vi "ControlEnhanced.vi"() -> ()   [LabVIEW 2018]
uses:
  <vilib>/Platform/TimedLoop/XDataNode/timing_clust.ctl
  <vilib>/Platform/TimedLoop/XDataNode/nitl_modes.ctl
  <vilib>/Platform/TimedLoop/XDataNode/wakeup.ctl
  <vilib>/myRIO/Instrument Drivers/Onboard IO/AI/typedefs/AI Reference.ctl
  <vilib>/myRIO/Common/Instrument Driver Framework/Utilities/typedefs/myRIO Generic Hardware Reference.ctl
  <vilib>/myRIO/Common/Instrument Driver Framework/Utilities/typedefs/Hardware Version Enum.ctl
  <vilib>/myRIO/Common/Instrument Driver Framework/Utilities/typedefs/myRIO v1.0 Reference.ctl
  <vilib>/myRIO/Common/Instrument Driver Framework/Utilities/typedefs/Generic FPGA Reference.ctl
  <vilib>/myRIO/Common/Instrument Driver Framework/myRIO v1.0/AI/typedefs/AI Channels List.ctl
  <vilib>/myRIO/Common/Instrument Driver Framework/myRIO v1.0/AI/typedefs/AI Channels Enum.ctl
  <vilib>/myRIO/Common/Instrument Driver Framework/Utilities/typedefs/Analog Scaling Constants List.ctl
  <vilib>/myRIO/Common/Instrument Driver Framework/Utilities/typedefs/Analog Scaling Constants.ctl
  <vilib>/userdefined/High Color/nirio_resource_hc.ctl
  <vilib>/myRIO/Instrument Drivers/Onboard IO/AO/typedefs/AO Reference.ctl
  <vilib>/myRIO/Common/Instrument Driver Framework/myRIO v1.0/AO/typedefs/AO Channels List.ctl
  <vilib>/myRIO/Common/Instrument Driver Framework/myRIO v1.0/AO/typedefs/AO Channels Enum.ctl
  <vilib>/myRIO/Common/Instrument Driver Framework/Utilities/vis/Is FPGA Ref Available.vi
  <vilib>/myRIO/Common/Instrument Driver Framework/myRIO v1.0/AI/vis/myRIO v1.1 Open AI.vi
  <vilib>/myRIO/Instrument Drivers/Onboard IO/AI/vis/Read.vi
  <vilib>/myRIO/Common/Instrument Driver Framework/myRIO v1.0/AO/vis/myRIO v1.1 Open AO.vi
  <vilib>/myRIO/Instrument Drivers/Onboard IO/AO/vis/Write.vi
  <vilib>/myRIO/Common/Instrument Driver Framework/myRIO v1.0/PWM/vis/myRIO v1.1 Open PWM.vi
  <vilib>/myRIO/Common/Instrument Driver Framework/Utilities/vis/Validate Channels.vi
  <vilib>/myRIO/Common/Instrument Driver Framework/myRIO v1.0/AI/vis/myRIO v1.0 Reserve AI.vi
  <vilib>/myRIO/Common/Instrument Driver Framework/myRIO v1.0/AO/vis/myRIO v1.0 Reserve AO.vi
  <vilib>/myRIO/Common/Instrument Driver Framework/myRIO v1.0/PWM/vis/myRIO v1.0 Reserve PWM.vi
  <vilib>/myRIO/Common/Instrument Driver Framework/myRIO v1.0/AI/vis/myRIO v1.0 Build MUX Configuration AI.vi
  <vilib>/myRIO/Common/Instrument Driver Framework/myRIO v1.0/Resource Manager/vis/myRIO v1.0 Reserve Channel List.vi
  <vilib>/myRIO/Common/Instrument Driver Framework/myRIO v1.0/AO/vis/myRIO v1.0 Build MUX Configuration AO.vi
  <vilib>/myRIO/Common/Instrument Driver Framework/myRIO v1.0/PWM/vis/myRIO v1.0 Build MUX Configuration PWM.vi
  <vilib>/myRIO/Common/Instrument Driver Framework/myRIO v1.0/Resource Manager/vis/myRIO v1.0 Reserve Channel.vi
  <vilib>/myRIO/Common/Instrument Driver Framework/myRIO v1.0/Resource Manager/vis/myRIO v1.0 Unreserve Channel.vi
  <vilib>/myRIO/Common/Instrument Driver Framework/myRIO v1.0/Resource Manager/vis/myRIO v1.0 Create Configuration List.vi
  <vilib>/myRIO/Common/Instrument Driver Framework/myRIO v1.0/Resource Manager/vis/myRIO v1.0 Build Mutex Name.vi
  <vilib>/Utility/VariantDataType/GetNumericInfo.vi
  <vilib>/Utility/error.llb/Error Cluster From Error Code.vi
  <vilib>/myRIO/Common/Instrument Driver Framework/myRIO v1.0/myRIO v1.1 Open.vi
  <vilib>/myRIO/Common/Instrument Driver Framework/myRIO v1.0/AI/vis/myRIO v1.0 Get Scaling Constants AI.vi
  <vilib>/myRIO/Common/Instrument Driver Framework/Utilities/vis/IO Manager.vi
  <vilib>/myRIO/Common/Instrument Driver Framework/Utilities/vis/Configuration Manager.vi
  <vilib>/myRIO/Common/Instrument Driver Framework/myRIO v1.0/myRIO v1.0 Close.vi
  <vilib>/myRIO/Common/Instrument Driver Framework/myRIO v1.0/AI/vis/myRIO v1.0 Read AI.vi
  <vilib>/myRIO/Common/Instrument Driver Framework/myRIO v1.0/AO/vis/myRIO v1.0 Get Scaling Constants AO.vi
  <vilib>/myRIO/Common/Instrument Driver Framework/myRIO v1.0/AO/vis/myRIO v1.0 Write AO.vi
  <vilib>/myRIO/Common/Instrument Driver Framework/myRIO v1.0/Resource Manager/vis/myRIO v1.0 Configure IO.vi
  <vilib>/myRIO/Common/Instrument Driver Framework/myRIO v1.0/PWM/vis/myRIO v1.0 Write PWM.vi
  <vilib>/platform/TimedLoop/XDataNode/XDataNode.xnode
  <vilib>/myRIO/Express VI/Onboard IO/AI/AI Express VI.xnode
  <vilib>/myRIO/Instrument Drivers/Onboard IO/AI/vis/myRIO AI Open.xnode
  <vilib>/myRIO/Express VI/Onboard IO/AO/AO Express VI.xnode
  <vilib>/myRIO/Instrument Drivers/Onboard IO/AO/vis/myRIO AO Open.xnode
  <vilib>/myRIO/Instrument Drivers/Onboard IO/AI/AI.lvlib
  <vilib>/myRIO/Instrument Drivers/Onboard IO/AO/AO.lvlib
  <vilib>/Platform/TimedLoop/XDataNode/XDNodeRunTimeDep.lvlib
  <vilib>/myRIO/Instrument Drivers/Onboard IO/PWM/PWM.lvlib
panel:
  in  "MAKE ACTUATOR EXPLODE":bool caption="Blank Button"
  out "FSR Voltage over Time":dbl(graph)
  in  "Stop Button":bool
  in  "Pressure \nSetpoint (kPa)":dbl(slide)=5.5 scale=0.0..30.0
  in  "PWM channel":tag="B/PWM0"
  in  "[ESC]":bool
  in  "Actuator Servo":dbl(slide) scale=-200.0..200.0
  in  "freq [Hz]":dbl=50.0
  out "pulse width [ms]":dbl=1.5
  out "duty cycle [%]":dbl
  in  "null offset":bool
  out "offset [%FS]":dbl
  in  "Button \nMode":bool
  out "bUTTON":bool
  out "Null Offset\n(Zero)":dbl
  in  "Ok":bool
  in  "Tolerance":dbl=0.5 format="%0.4f"
  in  "CRUSH IT":bool caption="Blank Button"
  in  "GRIP HARDER":bool caption="Blank Button"
  in  "GRIP":bool caption="Blank Button"
  in  "RELEASE":bool caption="Blank Button"
  in  "SoVal On/Off":bool
  in  "Gas Reg\n(Manual)":dbl(slide) scale=0.0..0.16
  in  "OK Button":bool
  in  "SELF-DESTRUCT BUTTON":bool
  in  "Operating Mode":string(combo)="1"
  in  "Upper \nBound":dbl=0.1 format="%#_13g"
  in  "Lower \nBound":dbl=0.04 format="%#_13g"
  in  "Signal Frequency / Hz":i64=200
  in  "Factor of Decrease":dbl=1e-05
  in  "Factor of Increase":dbl=1e-05
  out "SoVal":bool
  in  "BIGGER SELF-DESTRUCT BUTTON":bool
  out "SoVal\nSoVal (C/AO0 (AO0))":dbl
  out "Gas Reg. (A/AO0 (Pin 2))":dbl=0.04 min=0.04 max=0.1
  in  "Pressure \nSetpoint":dbl(slide)=5.5 scale=0.0..10.0
  out "Force Resistor kPa)":dbl
  out "FSR Dial (kPa)":dbl(knob) scale=-0.5..30.0
  out "PP 2":dbl
  out "PP Dial":dbl(knob) scale=-0.5..11.0
  out "PP":bool
  out "FSR":bool
  in  "PP Weight":dbl=0.1 min=0.0 max=1.0 step=0.001
  in  "FSR Weight":dbl=0.1 min=0.0 max=1.0 step=0.0001
  # "WARNING: it really does what it says."
  # "These are calculated based on the user-input lower and upper bounds. TODO: hide these buttons in automatic mode"
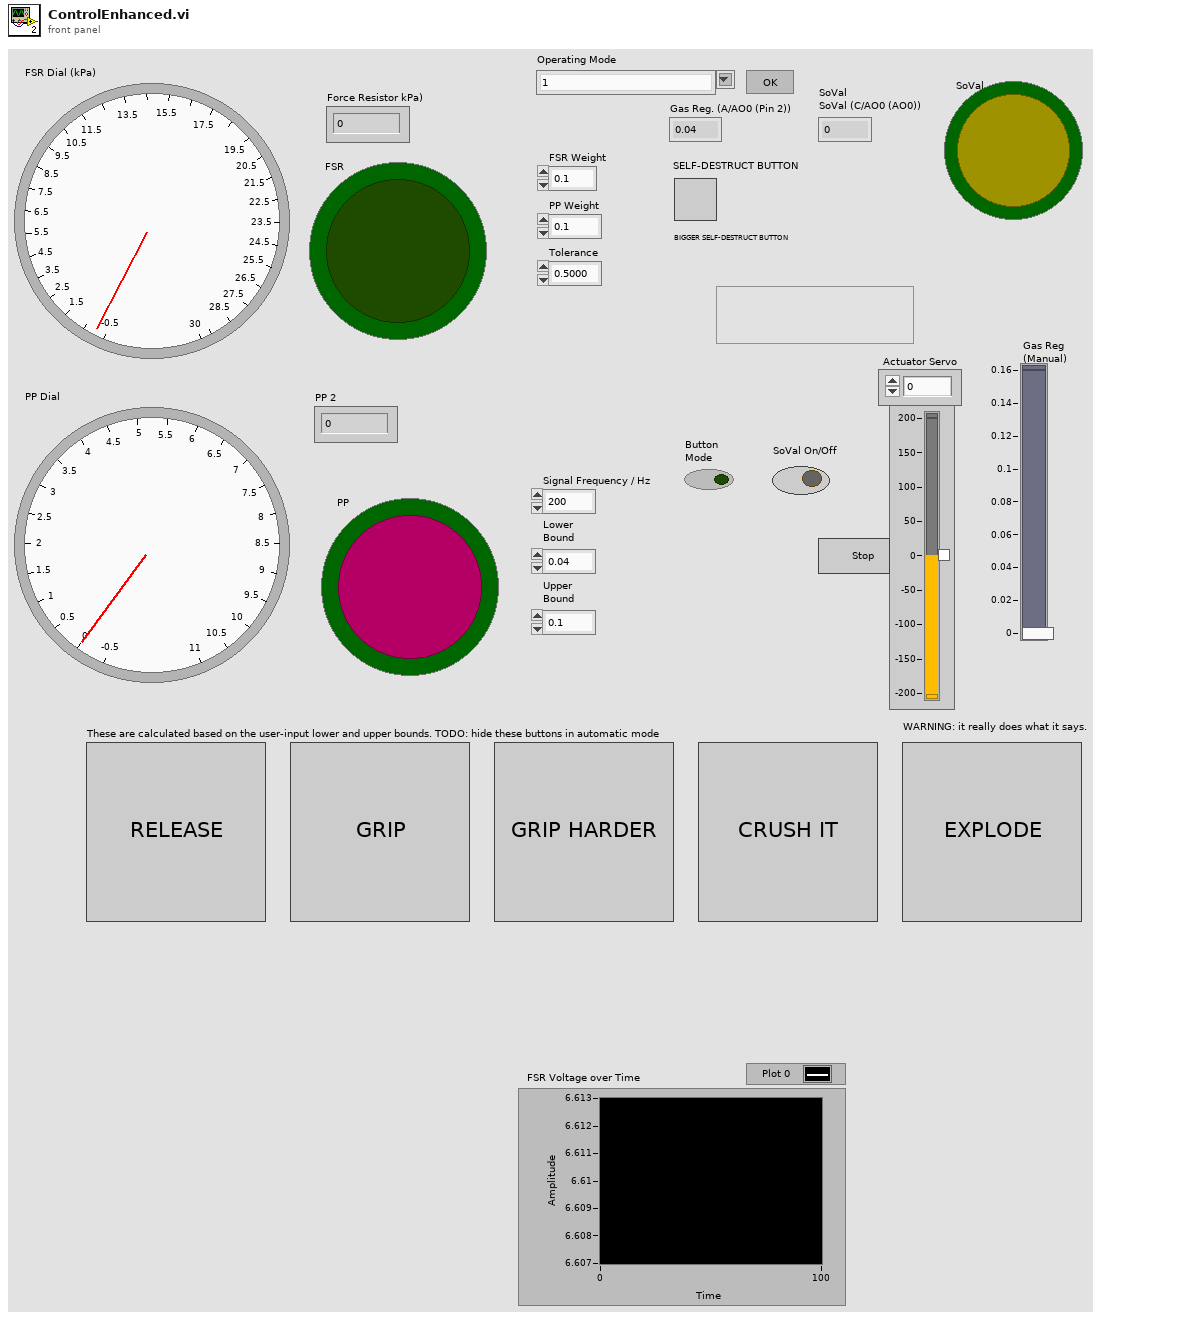
[diagram p1: front panel]
types:
  T1 = typedef "XDNodeRunTimeDep.lvlib/timing_clust.ctl" = cluster{"Expected End [f-1]":u64, "Actual End [f-1]":u64, "Finished Late? [f-1]":bool, "Expected End [i-1]":u64, "Actual End [i-1]":u64, "Finished Late? [i-1]":bool, "Expected Start [i]":u64, "Actual Start [i]":u64, "Expected Start [f]":u64, "Actual Start [f]":u64, "Source Name":string, "Structure Name":string, "Period":i64, "Deadline":i64, "Offset":i64, "Start":i64, "Priority":i32, "Timeout":i32, "Mode":T2, "Wakeup Reason":T3, "Error":errorcluster, "Source Type":string, "Secondary Source Type":string, "Global End Time":u64, "Global Start Time":u64, "Frame Duration":u64, "Iteration Duration":u64, "Assigned CPU":i32, "I/O Scan Engine Mode":u32}
  T2 = typedef "XDNodeRunTimeDep.lvlib/nitl_modes.ctl" = enum32{"No Change", "Process missed periods, maintain original phase", "Discard missed periods, maintain original phase", "Process missed periods, ignore original phase", "Discard missed periods, ignore original phase"}
  T3 = typedef "XDNodeRunTimeDep.lvlib/wakeup.ctl" = enum32{"Normal", "Aborted", "Asynchronous wakeup", "Timing source error", "Timed loop error", "Timeout"}
  T4 = typedef "AO.lvlib/AO Reference.ctl" = cluster{"myRIO Reference":T5, "AO Channel List":T9, "AO Scaling Constant List":T11}
  T5 = typedef "myRIO Generic Hardware Reference.ctl" = cluster{"myRIO Model":T6, "myRIO Hardware Reference":T7}
  T6 = typedef "Hardware Version Enum.ctl" = enum16{"Unknown", "myRIO-1900", "myRIO-1950", "roboRIO", "NI ELVIS RIO CM", "ELVIS III"}
  T7 = typedef "myRIO v1.0 Reference.ctl" = cluster{"Generic FPGA Reference":T8, "Allow multiple opens":bool}
  T8 = typedef "Generic FPGA Reference.ctl" = refnum<k20>
  T9 = typedef "AO Channels List.ctl" = T10[]
  T10 = typedef "AO Channels Enum.ctl" = enum16{"Not Connected", "AudioOut/Left", "AudioOut/Right", "C/AO0", "C/AO1", "A/AO0", "A/AO1", "B/AO0", "B/AO1"}
  T11 = typedef "Analog Scaling Constants List.ctl" = T12[]
  T12 = typedef "Analog Scaling Constants.ctl" = cluster{"LSB Weight (Volts)":dbl, "Offset (Volts)":dbl, "Signed?":bool}
  T13 = typedef "nirio_resource_hc.ctl" = tag
  T14 = typedef "AI.lvlib/AI Reference.ctl" = cluster{"myRIO Reference":T5, "AI Channels List":T15, "AI Scaling Constants List":T11}
  T15 = typedef "AI Channels List.ctl" = T16[]
  T16 = typedef "AI Channels Enum.ctl" = enum16{"Not Connected", "AudioIn/Left", "AudioIn/Right", "C/AI0", "C/AI1", "A/AI0", "A/AI1", "A/AI2", "A/AI3", "A/AI4", "A/AI5", "A/AI6", "A/AI7", "B/AI0", "B/AI1", "B/AI2", "B/AI3", "B/AI4", "B/AI5", "B/AI6", "B/AI7", "AI/AI0", "AI/AI1", "AI/AI2", "AI/AI3", "A/AI0 (DIFF)", "A/AI1 (DIFF)", "A/AI2 (DIFF)", "A/AI3 (DIFF)", "B/AI0 (DIFF)", "B/AI1 (DIFF)", "B/AI2 (DIFF)", "B/AI3 (DIFF)"}
  T17 = typedef "PWM.lvlib/PWM Reference.ctl" = cluster{"myRIO Reference":T5, "PWM Channels Enum":T18, "PWM Configuration":T19}
  T18 = typedef "PWM Channels Enum.ctl" = enum16{"Not Connected", "C/PWM0", "C/PWM1", "A/PWM0", "A/PWM1", "A/PWM2", "A/PWM3", "A/PWM4", "A/PWM5", "A/PWM6", "A/PWM7", "A/PWM8", "A/PWM9", "A/PWM10", "A/PWM11", "A/PWM12", "A/PWM13", "A/PWM14", "A/PWM15", "A/PWM16", "A/PWM17", "A/PWM18", "A/PWM19", "B/PWM0", "B/PWM1", "B/PWM2", "B/PWM3", "B/PWM4", "B/PWM5", "B/PWM6", "B/PWM7", "B/PWM8", "B/PWM9", "B/PWM10", "B/PWM11", "B/PWM12", "B/PWM13", "B/PWM14", "B/PWM15", "B/PWM16", "B/PWM17", "B/PWM18", "B/PWM19", "PWM/PWM0", "PWM/PWM1", "PWM/PWM2", "PWM/PWM3", "PWM/PWM4", "PWM/PWM5", "PWM/PWM6", "PWM/PWM7", "PWM/PWM8", "PWM/PWM9"}
  T19 = typedef "PWM.lvlib/PWM Configuration.ctl" = cluster{"Frequency":dbl, "Duty Cycle":dbl}
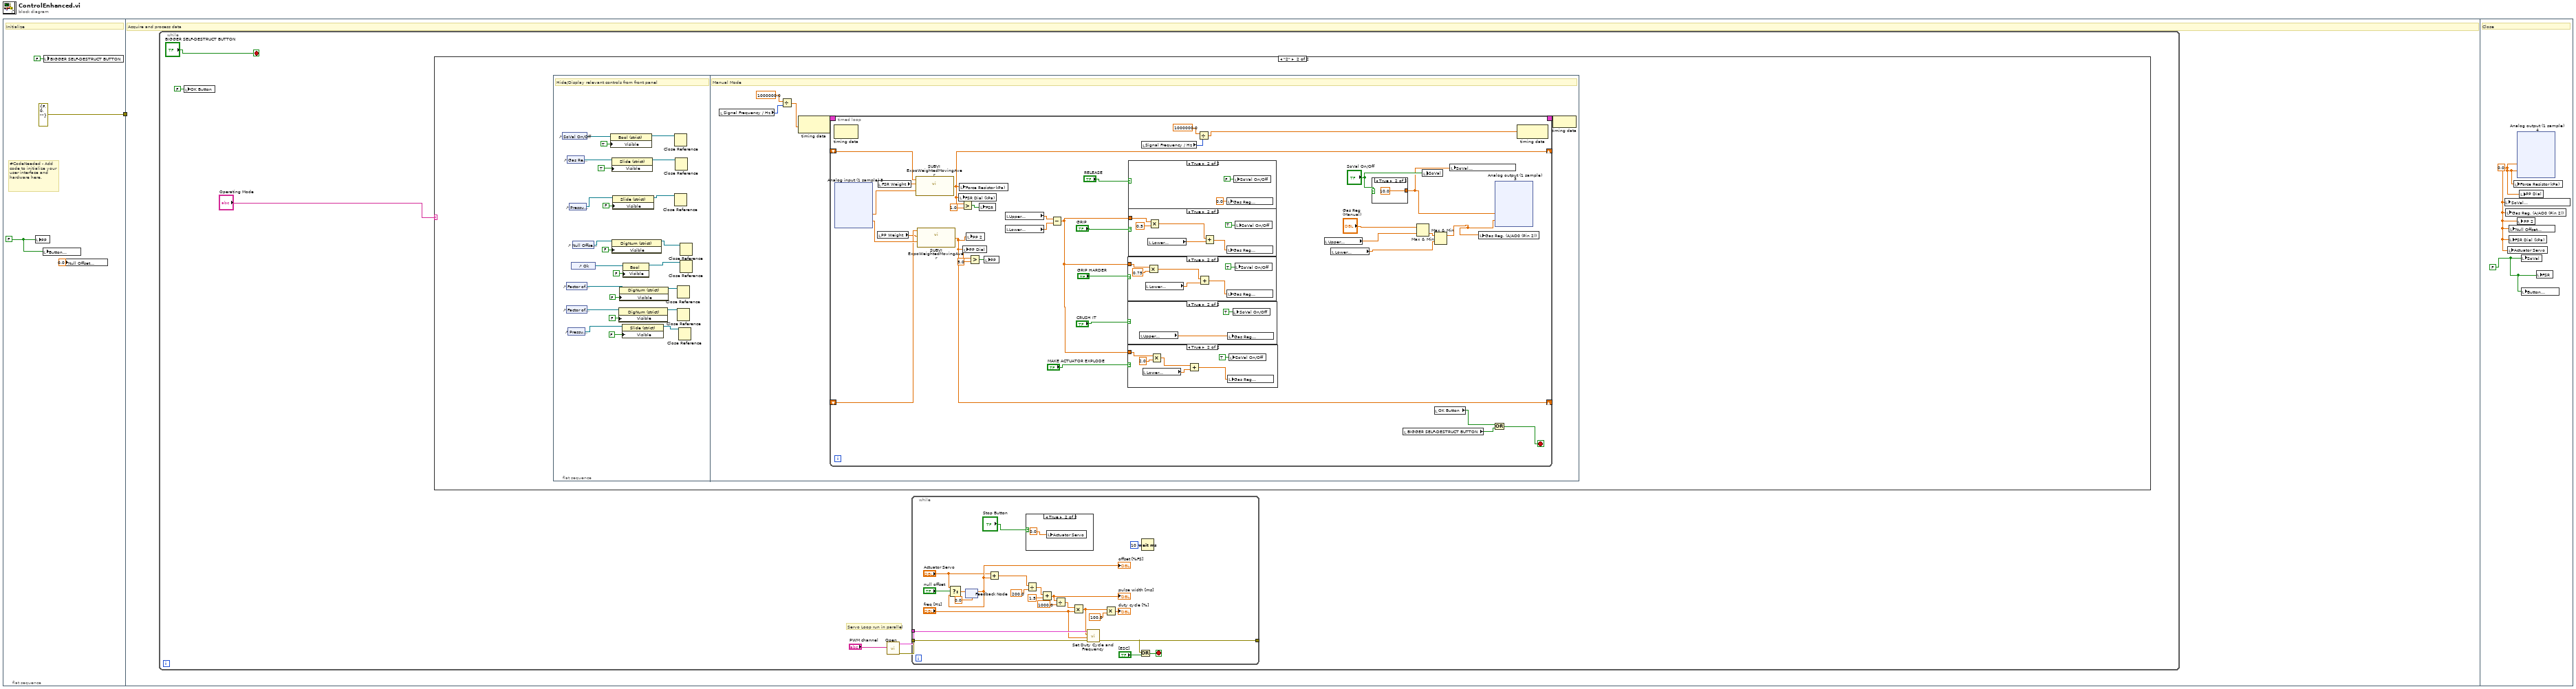
[diagram p0: block diagram]
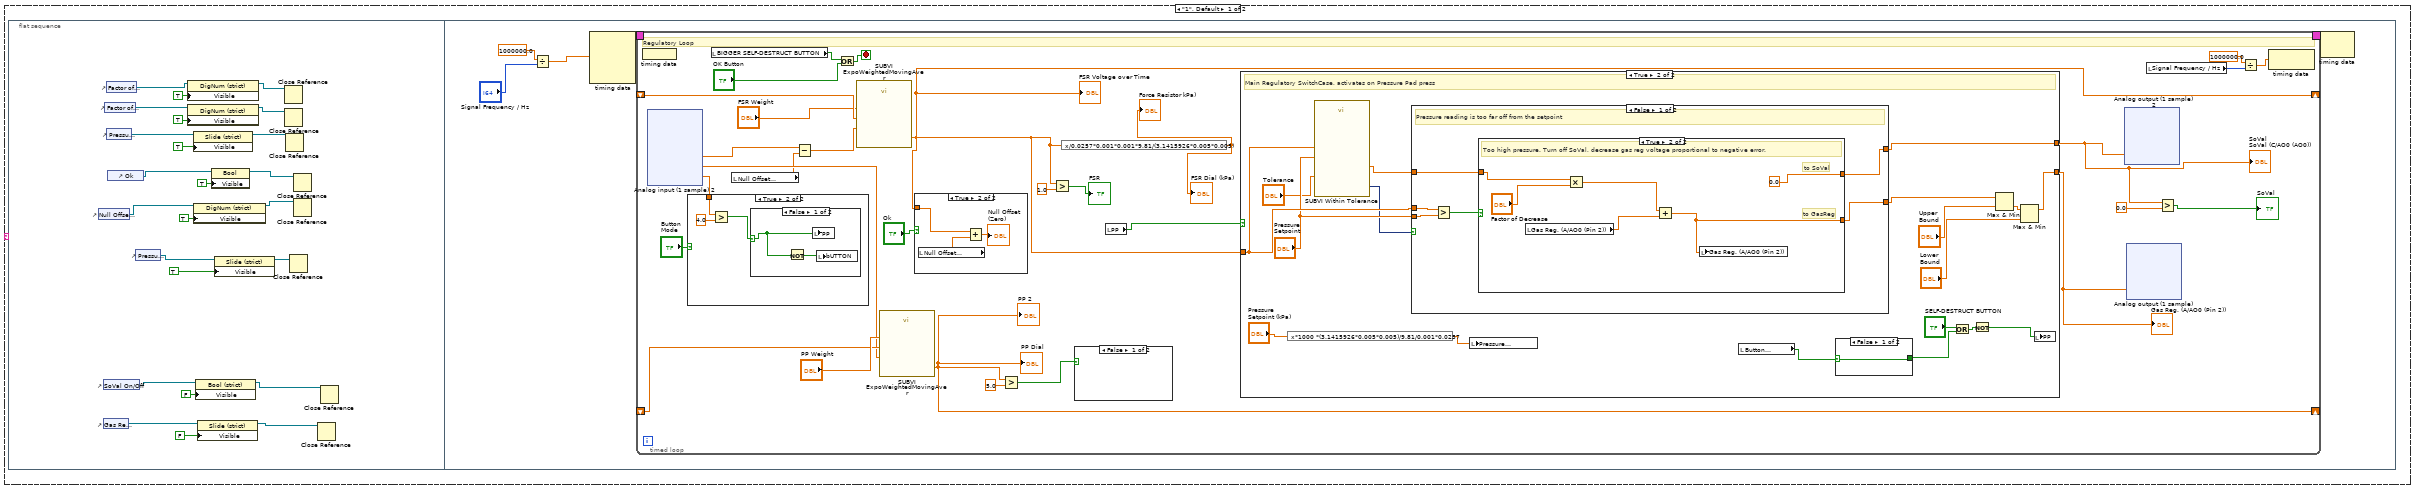
[diagram p3: hidden frame]
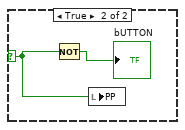
[diagram p5: hidden frame]
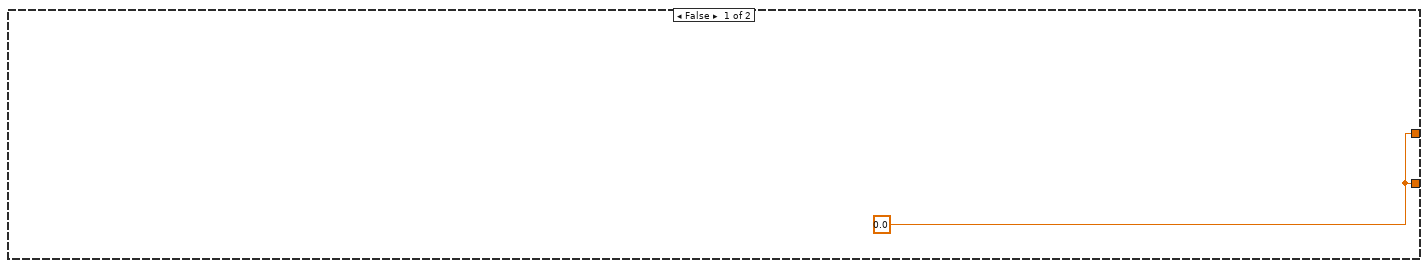
[diagram p7: hidden frame]
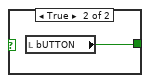
[diagram p8: hidden frame]
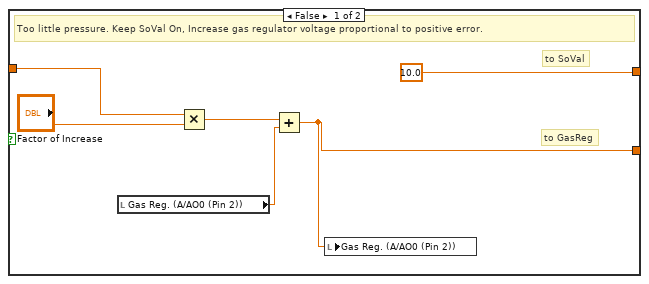
[diagram p9: hidden frame]
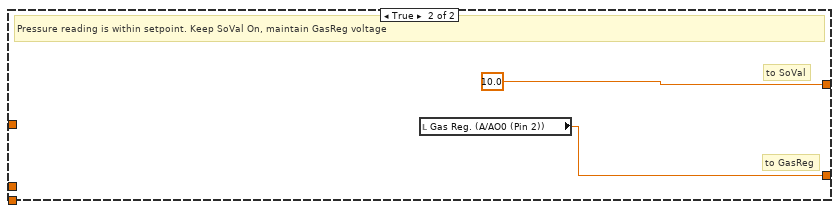
[diagram p10: hidden frame]
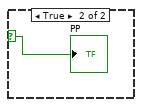
[diagram p11: hidden frame]
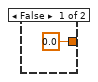
[diagram p17: hidden frame]
diagram:
  n1 = flat-sequence {
    tunnel: [errorcluster {"status"=FALSE, "code"=0, "source"=""} ("error in (no error)")] -> w1
    tunnel: w1 -> [_]
    frame #0 {
      w2 = FALSE ("PP")
      # "#CodeNeeded - Add code to initialize your user interface and hardware here."
      # "Initialize"
      n2 = local write "PP"(w2) -> ()
      n3 = local write "Button \nMode"(w2) -> ()
      n4 = local write "BIGGER SELF-DESTRUCT BUTTON"(FALSE ("BIGGER SELF-DESTRUCT BUTTON")) -> ()
      n5 = local write "Null Offset\n(Zero)"(0.0 ("Null Offset")) -> ()
    }
    frame #1 {
      # "Acquire and process data"
      n6 = while {
        stop <- "BIGGER SELF-DESTRUCT BUTTON" stop-if-true
        # "Servo Loop run in parallel"
        n7 = local write "OK Button"(FALSE ("OK Button")) -> ()
        n8 = case shown="\"2\"" "Operating Mode" {
          frame "1", Default {
            n9 = flat-sequence {
              frame #0 {
                n10 = control-ref of="Null Offset\n(Zero)"() -> (w41:refnum<vi>)
                n11 = control-ref of="Gas Reg\n(Manual)"() -> (w55:refnum<vi>)
                n12 = control-ref of="SoVal On/Off"() -> (w53:refnum<vi>)
                n13 = control-ref of="Factor of Decrease"() -> (w56:refnum<vi>)
                n14 = control-ref of="Factor of Increase"() -> (w59:refnum<vi>)
                n15 = control-ref of="Pressure \nSetpoint"() -> (w49:refnum<vi>)
                n16 = control-ref of="Ok"() -> (w42:refnum<vi>)
                n17 = control-ref of="Pressure \nSetpoint (kPa)"() -> (w37:refnum<vi>)
                n18 = property class="DigNum (strict)"(reference=w59, "Visible"=TRUE) -> (reference out=w57:refnum<vi>)  [unwired: 1 in, 1 out]
                n19 = property class="DigNum (strict)"(reference=w56, "Visible"=TRUE) -> (reference out=w58:refnum<vi>)  [unwired: 1 in, 1 out]
                n20 = property class="Slide (strict)"(reference=w49, "Visible"=TRUE) -> (reference out=w48:refnum<vi>)  [unwired: 1 in, 1 out]
                n21 = property class="DigNum (strict)"(reference=w41, "Visible"=TRUE) -> (reference out=w43:refnum<vi>)  [unwired: 1 in, 1 out]
                n22 = property class="Bool (strict)"(reference=w53, "Visible"=FALSE) -> (reference out=w52:refnum<vi>)  [unwired: 1 in, 1 out]
                n23 = property class="Slide (strict)"(reference=w55, "Visible"=FALSE) -> (reference out=w51:refnum<vi>)  [unwired: 1 in, 1 out]
                n24 = property class="Bool"(reference=w42, "Visible"=TRUE) -> (reference out=w44:refnum<vi>)  [unwired: 1 in, 1 out]
                n25 = property class="Slide (strict)"(reference=w37, "Visible"=TRUE) -> (reference out=w36:refnum<vi>)  [unwired: 1 in, 1 out]
                n26 = Close Reference(reference=w57) -> ()  [unwired: 1 in, 1 out]
                n27 = Close Reference(reference=w58) -> ()  [unwired: 1 in, 1 out]
                n28 = Close Reference(reference=w48) -> ()  [unwired: 1 in, 1 out]
                n29 = Close Reference(reference=w36) -> ()  [unwired: 1 in, 1 out]
                n30 = Close Reference(reference=w44) -> ()  [unwired: 1 in, 1 out]
                n31 = Close Reference(reference=w43) -> ()  [unwired: 1 in, 1 out]
                n32 = Close Reference(reference=w51) -> ()  [unwired: 1 in, 1 out]
                n33 = Close Reference(reference=w52) -> ()  [unwired: 1 in, 1 out]
              }
              frame #1 {
                n34 = Divide(x=1000000.0, y="Signal Frequency / Hz") -> (x/y=w62:dbl)
                n35 = node-c288(w62) -> (w64:T1)  [unwired: 3 in]
                n36 = timed-loop "Timed Loop" {
                  shift-right: [w88] -> _
                  shift-left: _ -> [w89]
                  shift-right: [w65] -> _
                  shift-left: _ -> [w87]
                  timing: w64 -> [_]
                  timing-out: [_] -> w63
                  stop <- w76 stop-if-true
                  # "Regulatory Loop"
                  n37 = node-c288() -> ()  [unwired: 1 in]
                  n38 = xnode "Analog input (1 sample) 2"() -> ("FSR (C/AI0 (AI0))"=w70:dbl, "PressurePad (C/AI1 (AI1))"=w74:dbl, "Button (A/AI0 (Pin 3))"=w68:dbl)  [unwired: 1 in, 1 out]
                  n39 = case shown="True" "Button \nMode" {
                    tunnel: w68 -> [_ w96]
                    frame False {
                    }
                    frame True {
                      n40 = Greater?(x=w96, y=4.0) -> (0:w94:bool)
                      n41 = case shown="False" w94 {
                        selector: w94 -> [w98 w99]
                        frame False {
                          n42 = Not(x=w98) -> (.not. x?=w97:bool)
                          n43 = local write "PP"(w98) -> ()
                          n44 = local write "bUTTON"(w97) -> ()
                        }
                        frame True {
                          n45 = Not(x=w99) -> (.not. x?=→"bUTTON":bool)
                          n46 = local write "PP"(w99) -> ()
                        }
                      }
                    }
                  }
                  n47 = local read "BIGGER SELF-DESTRUCT BUTTON"() -> (w77:bool)
                  n48 = local read "Null Offset\n(Zero)"() -> (w69:dbl)
                  n49 = Subtract(x=w70, y=w69) -> (x-y=w71:dbl)
                  n50 = Or(x=w77, y="OK Button") -> (x .or. y?=w76:bool)
                  n51 = call "SUBVI ExpoWeightedMovingAver.vi"("New Sample"=w71, "EWMA Weight"="FSR Weight", "Old Estimate"=w87) -> ("Weighted Average"=w65:dbl)  [unwired: 8 in]
                  "FSR Voltage over Time" <- w65
                  n52 = call "SUBVI ExpoWeightedMovingAver.vi"("New Sample"=w74, "EWMA Weight"="PP Weight", "Old Estimate"=w89) -> ("Weighted Average"=w88:dbl)  [unwired: 8 in]
                  "PP 2" <- w88
                  "PP Dial" <- w88
                  n53 = case shown="True" "Ok" {
                    tunnel: w65 -> [_ w103]
                    frame False {
                    }
                    frame True {
                      n54 = local read "Null Offset\n(Zero)"() -> (w101:dbl)
                      n55 = Add(x=w103, y=w101) -> (x+y=→"Null Offset\n(Zero)":dbl)
                    }
                  }
                  n56 = Greater?(x=w88, y=5.0) -> (0:w85:bool)
                  n57 = Greater?(x=w65, y=1.0) -> (0:→"FSR":bool)
                  n58 = expression code="x/0.0257*0.001*0.001*9.81/(3.1415926*0.005*0.005)"(w65) -> (→"Force Resistor kPa)" →"FSR Dial (kPa)":dbl)
                  n59 = case shown="False" w85 {
                    selector: w85 -> [_ w223]
                    frame False {
                    }
                    frame True {
                      "PP" <- w223
                    }
                  }
                  n60 = local read "PP"() -> (w84:bool)
                  n61 = case shown="True" w84 {
                    tunnel: w65 -> [_ w193]
                    tunnel: [w182 w195] -> w83
                    tunnel: [w182 w198] -> w73
                    frame False {
                      w182 = 0.0
                    }
                    frame True {
                      # "Main Regulatory SwitchCase, activates on Pressure Pad press"
                      n62 = expression code="x*1000 *(3.1415926*0.005*0.005)/9.81/0.001*0.0257"("Pressure \nSetpoint (kPa)") -> (w184:dbl)
                      n63 = call "SUBVI Within Tolerance.vi"("Constant Value to Compare Against"="Pressure \nSetpoint", "Tol"="Tolerance", "Operand 1"=w193) -> ("Discrepancy"=w183:dbl, "Result"=w191:dynamicdata)  [unwired: 6 in, 1 out]
                      n64 = case shown="False" w191 {
                        tunnel: [w205 w222] -> w200
                        tunnel: w193 -> [w208 _]
                        tunnel: "Pressure \nSetpoint" -> [w207 _]
                        tunnel: [w204 10.0 ("SoVal\nSoVal (C/AO0 (AO0))")] -> w198
                        tunnel: w183 -> [w203 _]
                        frame False {
                          # "Pressure reading is too far off from the setpoint"
                          n65 = Greater?(x=w208, y=w207) -> (0:w206:bool)
                          n66 = case shown="True" w206 {
                            tunnel: [w214 w220] -> w205
                            tunnel: [10.0 0.0] -> w204
                            tunnel: w203 -> [w210 w218]
                            frame False {
                              # "to GasReg"
                              # "to SoVal"
                              # "Too little pressure. Keep SoVal On, Increase gas regulator voltage proportional to positive error."
                              n67 = local read "Gas Reg. (A/AO0 (Pin 2))"() -> (w212:dbl)
                              n68 = Multiply(x=w210, y="Factor of Increase") -> (x*y=w209:dbl)
                              n69 = Add(x=w209, y=w212) -> (x+y=w214:dbl)
                              n70 = local write "Gas Reg. (A/AO0 (Pin 2))"(w214) -> ()
                            }
                            frame True {
                              # "to GasReg"
                              # "to SoVal"
                              # "Too high pressure. Turn off SoVal, decrease gas reg voltage proportional to negative error."
                              n71 = local read "Gas Reg. (A/AO0 (Pin 2))"() -> (w216:dbl)
                              n72 = Multiply(x=w218, y="Factor of Decrease") -> (x*y=w215:dbl)
                              n73 = Add(x=w215, y=w216) -> (x+y=w220:dbl)
                              n74 = local write "Gas Reg. (A/AO0 (Pin 2))"(w220) -> ()
                            }
                          }
                        }
                        frame True {
                          # "to GasReg"
                          # "to SoVal"
                          # "Pressure reading is within setpoint. Keep SoVal On, maintain GasReg voltage"
                          n75 = local read "Gas Reg. (A/AO0 (Pin 2))"() -> (w222:dbl)
                        }
                      }
                      n76 = local write "Pressure \nSetpoint"(w184) -> ()
                      n77 = local read "Button \nMode"() -> (w186:bool)
                      n78 = case shown="False" w186 {
                        selector: w186 -> [w201 _]
                        tunnel: [w201 w202] -> w188
                        frame False {
                        }
                        frame True {
                          n79 = local read "bUTTON"() -> (w202:bool)
                        }
                      }
                      n80 = Or(x="SELF-DESTRUCT BUTTON", y=w188) -> (x .or. y?=w187:bool)
                      n81 = Not(x=w187) -> (.not. x?=w194:bool)
                      n82 = Max & Min(x=w200, y="Upper \nBound") -> (min(x,y)=w197:dbl)  [unwired: 1 out]
                      n83 = Max & Min(x=w197, y="Lower \nBound") -> (max(x,y)=w195:dbl)  [unwired: 1 out]
                      n84 = local write "PP"(w194) -> ()
                    }
                  }
                  "Gas Reg. (A/AO0 (Pin 2))" <- w83
                  "SoVal\nSoVal (C/AO0 (AO0))" <- w73
                  n85 = xnode "Analog output (1 sample) 2"("SoVal (C/AO0 (AO0))"=w73) -> ()  [unwired: 1 in, 1 out]
                  n86 = xnode "Analog output (1 sample)"("Gas Reg. (A/AO0 (Pin 2))"=w83) -> ()  [unwired: 1 in, 1 out]
                  n87 = local read "Signal Frequency / Hz"() -> (w79:i64)
                  n88 = Greater?(x=w73, y=0.0) -> (0:→"SoVal":bool)
                  n89 = Divide(x=1000000.0, y=w79) -> (x/y=w78:dbl)
                  n90 = node-c288(w78) -> ()  [unwired: 1 out]
                }
                n91 = node-c288(w63) -> ()  [unwired: 1 out]
              }
            }
          }
          frame "2" {
            n92 = flat-sequence {
              frame #0 {
                # "Hide/Display relevant controls from front panel"
                n93 = control-ref of="SoVal On/Off"() -> (w290:refnum<vi>)
                n94 = control-ref of="Factor of Increase"() -> (w283:refnum<vi>)
                n95 = control-ref of="Factor of Decrease"() -> (w285:refnum<vi>)
                n96 = control-ref of="Gas Reg\n(Manual)"() -> (w289:refnum<vi>)
                n97 = control-ref of="Pressure \nSetpoint"() -> (w286:refnum<vi>)
                n98 = control-ref of="Pressure \nSetpoint (kPa)"() -> (w269:refnum<vi>)
                n99 = control-ref of="Ok"() -> (w273:refnum<vi>)
                n100 = control-ref of="Null Offset\n(Zero)"() -> (w272:refnum<vi>)
                n101 = property class="Bool (strict)"(reference=w290, "Visible"=TRUE) -> (reference out=w287:refnum<vi>)  [unwired: 1 in, 1 out]
                n102 = property class="Slide (strict)"(reference=w289, "Visible"=TRUE) -> (reference out=w288:refnum<vi>)  [unwired: 1 in, 1 out]
                n103 = property class="DigNum (strict)"(reference=w272, "Visible"=FALSE) -> (reference out=w274:refnum<vi>)  [unwired: 1 in, 1 out]
                n104 = property class="Slide (strict)"(reference=w269, "Visible"=FALSE) -> (reference out=w267:refnum<vi>)  [unwired: 1 in, 1 out]
                n105 = property class="DigNum (strict)"(reference=w285, "Visible"=FALSE) -> (reference out=w284:refnum<vi>)  [unwired: 1 in, 1 out]
                n106 = property class="DigNum (strict)"(reference=w283, "Visible"=FALSE) -> (reference out=w282:refnum<vi>)  [unwired: 1 in, 1 out]
                n107 = property class="Slide (strict)"(reference=w286, "Visible"=FALSE) -> (reference out=w276:refnum<vi>)  [unwired: 1 in, 1 out]
                n108 = property class="Bool"(reference=w273, "Visible"=FALSE) -> (reference out=w275:refnum<vi>)  [unwired: 1 in, 1 out]
                n109 = Close Reference(reference=w267) -> ()  [unwired: 1 in, 1 out]
                n110 = Close Reference(reference=w287) -> ()  [unwired: 1 in, 1 out]
                n111 = Close Reference(reference=w288) -> ()  [unwired: 1 in, 1 out]
                n112 = Close Reference(reference=w282) -> ()  [unwired: 1 in, 1 out]
                n113 = Close Reference(reference=w284) -> ()  [unwired: 1 in, 1 out]
                n114 = Close Reference(reference=w276) -> ()  [unwired: 1 in, 1 out]
                n115 = Close Reference(reference=w274) -> ()  [unwired: 1 in, 1 out]
                n116 = Close Reference(reference=w275) -> ()  [unwired: 1 in, 1 out]
              }
              frame #1 {
                # "Manual Mode"
                n117 = local read "Signal Frequency / Hz"() -> (w293:i64)
                n118 = Divide(x=1000000.0, y=w293) -> (x/y=w291:dbl)
                n119 = node-c288(w291) -> (w295:T1)
                n120 = timed-loop {
                  timing: w295 -> [_]
                  timing-out: [_] -> w294
                  shift-right: [w319] -> _
                  shift-left: _ -> [w323]
                  shift-right: [w316] -> _
                  shift-left: _ -> [w322]
                  stop <- w310 stop-if-true
                  n121 = node-c288() -> ()  [unwired: 1 in, 1 out]
                  n122 = xnode "Analog input (1 sample) 3"() -> ("FSR (C/AI0 (AI0))"=w325:dbl, "PressurePad (C/AI1 (AI1))"=w324:dbl)  [unwired: 1 in, 1 out]
                  n123 = local read "PP Weight"() -> (w320:dbl)
                  n124 = local read "FSR Weight"() -> (w321:dbl)
                  n125 = call "SUBVI ExpoWeightedMovingAver.vi"("New Sample"=w325, "EWMA Weight"=w321, "Old Estimate"=w323) -> ("Weighted Average"=w319:dbl)  [unwired: 8 in]
                  n126 = call "SUBVI ExpoWeightedMovingAver.vi"("New Sample"=w324, "EWMA Weight"=w320, "Old Estimate"=w322) -> ("Weighted Average"=w316:dbl)  [unwired: 8 in]
                  n127 = local write "FSR Dial (kPa)"(w319) -> ()
                  n128 = local write "Force Resistor kPa)"(w319) -> ()
                  n129 = Greater?(x=w319, y=1.0) -> (0:w318:bool)
                  n130 = local write "PP Dial"(w316) -> ()
                  n131 = local write "PP 2"(w316) -> ()
                  n132 = Greater?(x=w316, y=5.0) -> (0:w315:bool)
                  n133 = local write "FSR"(w318) -> ()
                  n134 = local write "PP"(w315) -> ()
                  n135 = local read "Upper \nBound"() -> (w299:dbl)
                  n136 = local read "Lower \nBound"() -> (w298:dbl)
                  n137 = Subtract(x=w299, y=w298) -> (x-y=w297:dbl)
                  n138 = case shown="True" "GRIP HARDER" {
                    tunnel: w297 -> [_ w341]
                    frame False {
                    }
                    frame True {
                      n139 = local read "Lower \nBound"() -> (w338:dbl)
                      n140 = Multiply(x=w341, y=0.75) -> (x*y=w339:dbl)
                      n141 = Add(x=w339, y=w338) -> (x+y=w337:dbl)
                      n142 = local write "Gas Reg\n(Manual)"(w337) -> ()
                      n143 = local write "SoVal On/Off"(TRUE ("SoVal On/Off")) -> ()
                    }
                  }
                  n144 = case shown="True" "CRUSH IT" {
                    frame False {
                    }
                    frame True {
                      n145 = local read "Upper \nBound"() -> (w335:dbl)
                      n146 = local write "Gas Reg\n(Manual)"(w335) -> ()
                      n147 = local write "SoVal On/Off"(TRUE ("SoVal On/Off")) -> ()
                    }
                  }
                  n148 = case shown="True" "MAKE ACTUATOR EXPLODE" {
                    tunnel: w297 -> [_ w333]
                    frame False {
                    }
                    frame True {
                      n149 = local read "Lower \nBound"() -> (w330:dbl)
                      n150 = Multiply(x=w333, y=2.0) -> (x*y=w331:dbl)
                      n151 = Add(x=w331, y=w330) -> (x+y=w329:dbl)
                      n152 = local write "Gas Reg\n(Manual)"(w329) -> ()
                      n153 = local write "SoVal On/Off"(TRUE ("SoVal On/Off")) -> ()
                    }
                  }
                  n154 = case shown="True" "RELEASE" {
                    frame False {
                    }
                    frame True {
                      n155 = local write "Gas Reg\n(Manual)"(0.0 ("Gas Reg\n(Manual)")) -> ()
                      n156 = local write "SoVal On/Off"(FALSE ("SoVal On/Off")) -> ()
                    }
                  }
                  n157 = case shown="True" "GRIP" {
                    tunnel: w297 -> [_ w347]
                    frame False {
                    }
                    frame True {
                      n158 = local read "Lower \nBound"() -> (w344:dbl)
                      n159 = Multiply(x=w347, y=0.5) -> (x*y=w345:dbl)
                      n160 = Add(x=w345, y=w344) -> (x+y=w343:dbl)
                      n161 = local write "Gas Reg\n(Manual)"(w343) -> ()
                      n162 = local write "SoVal On/Off"(TRUE ("SoVal On/Off")) -> ()
                    }
                  }
                  n163 = local read "Signal Frequency / Hz"() -> (w327:i64)
                  n164 = Divide(x=1000000.0, y=w327) -> (x/y=w326:dbl)
                  n165 = local read "Upper \nBound"() -> (w306:dbl)
                  n166 = local read "Lower \nBound"() -> (w305:dbl)
                  n167 = case shown="True" "SoVal On/Off" {
                    tunnel: [0.0 10.0] -> w309
                    frame False {
                    }
                    frame True {
                    }
                  }
                  n168 = local read "BIGGER SELF-DESTRUCT BUTTON"() -> (w311:bool)
                  n169 = Max & Min(x="Gas Reg\n(Manual)", y=w306) -> (min(x,y)=w308:dbl)  [unwired: 1 out]
                  n170 = local write "SoVal"("SoVal On/Off") -> ()
                  n171 = Max & Min(x=w308, y=w305) -> (max(x,y)=w304:dbl)  [unwired: 1 out]
                  n172 = local read "OK Button"() -> (w312:bool)
                  n173 = local write "SoVal\nSoVal (C/AO0 (AO0))"(w309) -> ()
                  n174 = local write "Gas Reg. (A/AO0 (Pin 2))"(w304) -> ()
                  n175 = Or(x=w312, y=w311) -> (x .or. y?=w310:bool)
                  n176 = xnode "Analog output (1 sample) 3"("SoVal (C/AO0 (AO0))"=w309, "Gas Reg (A/AO0 (Pin 2))"=w304) -> ()  [unwired: 1 in, 1 out]
                  n177 = node-c288(w326) -> ()  [unwired: 1 out]
                }
                n178 = node-c288(w294) -> ()
              }
            }
          }
        }
        n179 = call <vilib>:"Open.vi"("Channel Name"="PWM channel") -> ("error out"=w8:errorcluster, "PWM Ref Out"=w7:T17)  [unwired: 9 in]
        n180 = while {
          tunnel: w7 -> [w26]
          tunnel: w8 -> [w25]
          tunnel: [w23] -> _
          stop <- w34 stop-if-true
          n181 = feedback #1(0.0 ("position [%FS]")) -> (w19:dbl)
          "offset [%FS]" <- w19
          n182 = Select(t="Actuator Servo", s="null offset", f=w19) -> (s? t:f=w21:dbl)
          n183 = feedback-in #1(w21) -> ()
          n184 = Add(x="Actuator Servo", y=w19) -> (x+y=w20:dbl)
          n185 = case shown="True" "Stop Button" {
            frame False {
            }
            frame True {
              n186 = local write "Actuator Servo"(0.0) -> ()
            }
          }
          n187 = Divide(x=w20, y=200.0) -> (x/y=w30:dbl)
          n188 = Add(x=w30, y=1.5) -> (x+y=w28:dbl)
          "pulse width [ms]" <- w28
          n189 = Divide(x=w28, y=1000.0) -> (x/y=w17:dbl)
          n190 = Multiply(x=w17, y="freq [Hz]") -> (x*y=w14:dbl)
          n191 = call <vilib>:"Set Duty Cycle and Frequency.vi"("error in (no error)"=w25, "Frequency [Hz]"="freq [Hz]", "Duty Cycle"=w14, "PWM Ref In"=w26) -> ("error out"=w23:errorcluster)  [unwired: 5 in, 1 out]
          n192 = Multiply(x=w14, y=100.0) -> (x*y=→"duty cycle [%]":dbl)
          n193 = Or(x=w23, y="[ESC]") -> (x .or. y?=w34:bool)
          n194 = Wait (ms)(milliseconds to wait=u32 10) -> ()  [unwired: 1 out]
        }
      }
    }
    frame #2 {
      w438 = FALSE
      w437 = 0.0
      # "Close"
      n195 = local write "SoVal\nSoVal (C/AO0 (AO0))"(w437) -> ()
      n196 = local write "Gas Reg. (A/AO0 (Pin 2))"(w437) -> ()
      n197 = local write "Actuator Servo"(w437) -> ()
      n198 = local write "FSR Dial (kPa)"(w437) -> ()
      n199 = local write "Null Offset\n(Zero)"(w437) -> ()
      n200 = local write "Force Resistor kPa)"(w437) -> ()
      n201 = local write "PP 2"(w437) -> ()
      n202 = xnode "Analog output (1 sample) 4"("C/AO0 (AO0)"=w437, "A/AO0 (Pin 2)"=w437) -> ()  [unwired: 1 in, 1 out]
      n203 = local write "PP Dial"(w437) -> ()
      n204 = local write "SoVal"(w438) -> ()
      n205 = local write "Button \nMode"(w438) -> ()
      n206 = local write "FSR"(w438) -> ()
    }
  }
